vi "Ch_data_title_pattern (SubVI).vi"(9 "Единица измерений":string) -> (0 "error out":errorcluster, 2 "Path":path, 3 "Byte Stream File out":refnum<file>, 6 "cancelled":bool)   [LabVIEW 2015]
panel:
  in  "error in":errorcluster
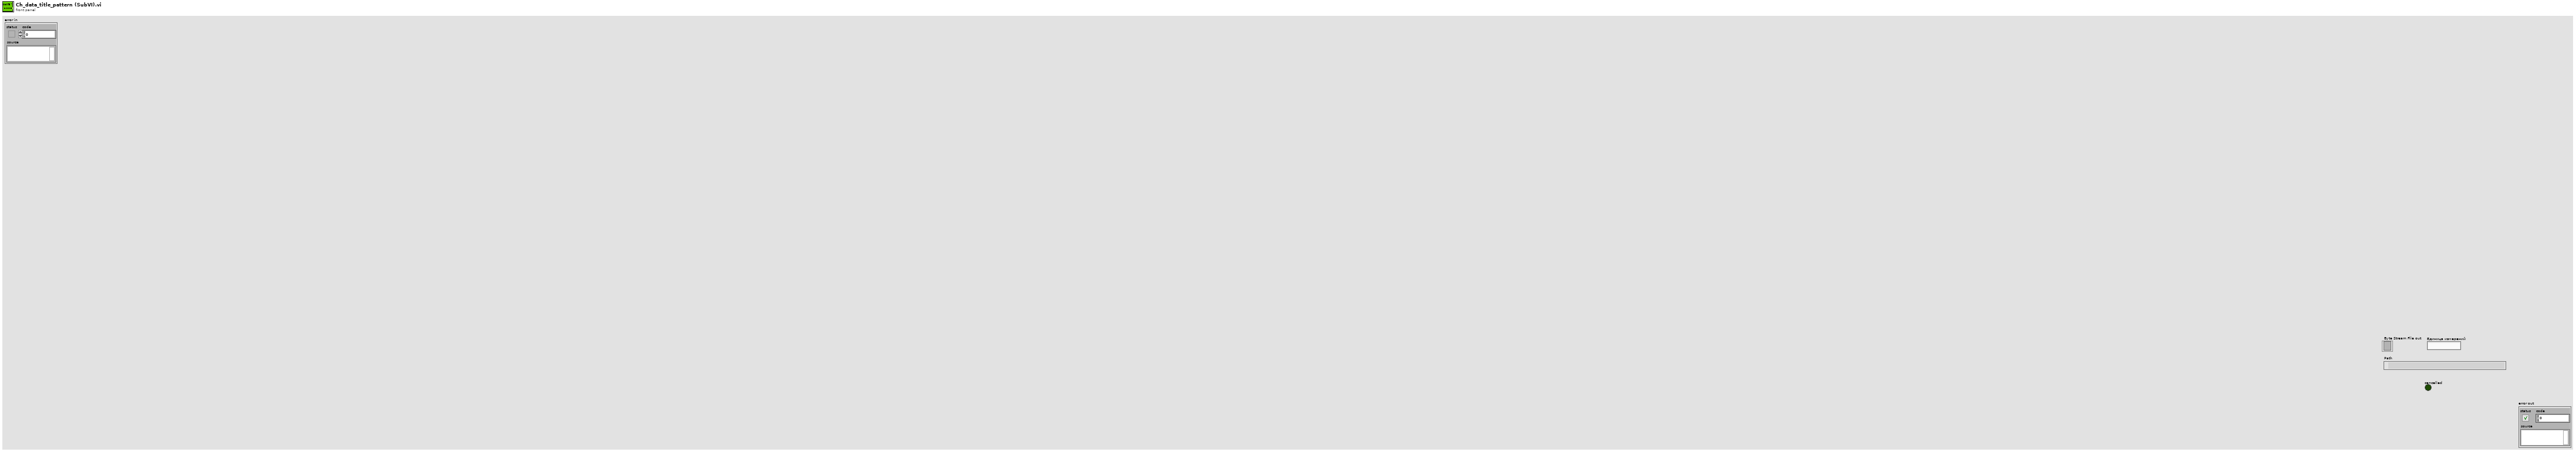
[diagram p1: front panel]
types:
  T1 = enum16{"open", "replace", "create", "open or create", "replace or create", "replace or create with confirmation"}
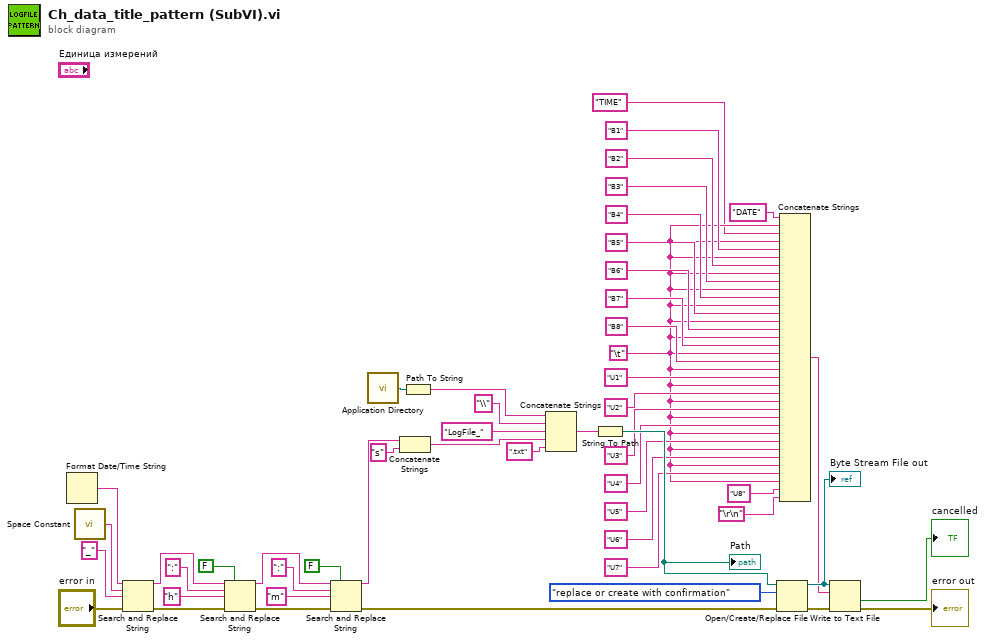
[diagram p0: block diagram]
diagram:
  w2 = "\t"
  n1 = Format Date/Time String() -> (date/time string=w46:string)  [unwired: 3 out]
  n2 = call <vilib>:"Space Constant.vi"() -> ("String"=w27:string)
  n3 = Search and Replace String(input string=w46, search string=w27, replace string="_" ("replace string (\"\")"), error in="error in") -> (result string=w29:string, error out=w39:errorcluster)  [unwired: 6 out]
  n4 = Search and Replace String(replace all?=FALSE ("replace all? (F)"), input string=w29, search string=":", replace string="h" ("replace string (\"\")"), error in=w39) -> (result string=w36:string, error out=w40:errorcluster)  [unwired: 5 out]
  n5 = Search and Replace String(replace all?=FALSE ("replace all? (F)"), input string=w36, search string=":", replace string="m" ("replace string (\"\")"), error in=w40) -> (result string=w41:string, error out=w25:errorcluster)  [unwired: 5 out]
  n6 = call <vilib>:"Application Directory.vi"() -> ("Application Directory"=w14:path)
  n7 = Concatenate Strings(w41, "s" ("string")) -> (w44:string)
  n8 = Path To String(path=w14) -> (string=w37:string)
  n9 = Concatenate Strings(w37, "\\" ("string"), "LogFile_" ("string"), w44, ".txt" ("default name")) -> (w26:string)
  n10 = String To Path(string=w26) -> (path=w24:path)
  "Path" <- w24
  n11 = Open/Create/Replace File(file path (use dialog)=w24, error in=w25, operation (0:open)=T1."replace or create with confirmation") -> (refnum out=w50:refnum<file>, error out=w48:errorcluster)  [unwired: 4 out]
  "Byte Stream File out" <- w50
  n12 = Concatenate Strings("DATE" ("string"), w2, "TIME" ("string"), w2, "B1" ("string"), w2, "B2" ("string"), w2, "B3" ("string"), w2, "B4" ("string"), w2, "B5" ("string"), w2, "B6" ("string"), w2, "B7" ("string"), w2, "B8" ("string"), w2, "U1" ("string"), w2, "U2" ("string"), w2, "U3" ("string"), w2, "U4" ("string"), w2, "U5" ("string"), w2, "U6" ("string"), w2, "U7" ("string"), w2, "U8" ("string"), "\r\n") -> (w47:string)
  n13 = Write to Text File(file (use dialog)=w50, text=w47, error in=w48) -> (cancelled=→"cancelled":bool, error out=→"error out":errorcluster)  [unwired: 2 out]
